vi "Generate Random Waveform.vi"(8 "error in":errorcluster, 11 "WaveformGen Settings":T1(array[cluster])) -> (0 "error out":errorcluster, 3 "Waveforms":waveform(dbl)[](array[waveform]))   [LabVIEW 2014]
uses:
  <userlib>/_OpenG.lib/numeric/numeric.llb/Random Number Within Range - DBL__ogtk.vi
  <vilib>/measure/NI_MABase.lvlib
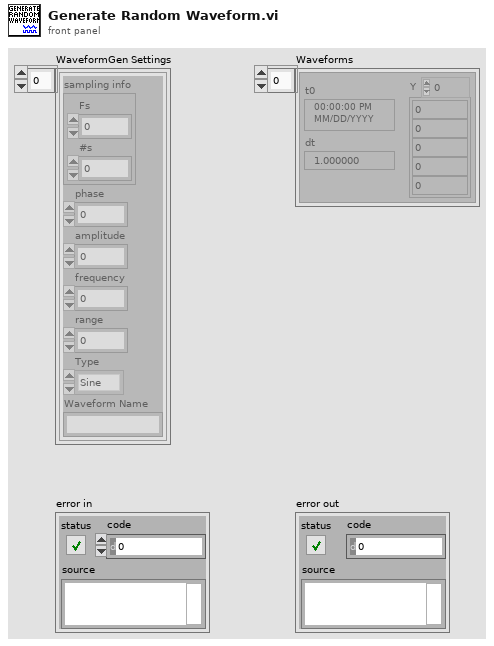
[diagram p1: front panel]
types:
  T1 = cluster{"sampling info":cluster{"Fs":dbl, "#s":dbl}, "phase":dbl, "amplitude":dbl, "frequency":dbl, "range":dbl, "Type":enum16{"Sine", "Triangle", "Sawtooth", "Square"}, "Waveform Name":string}[]
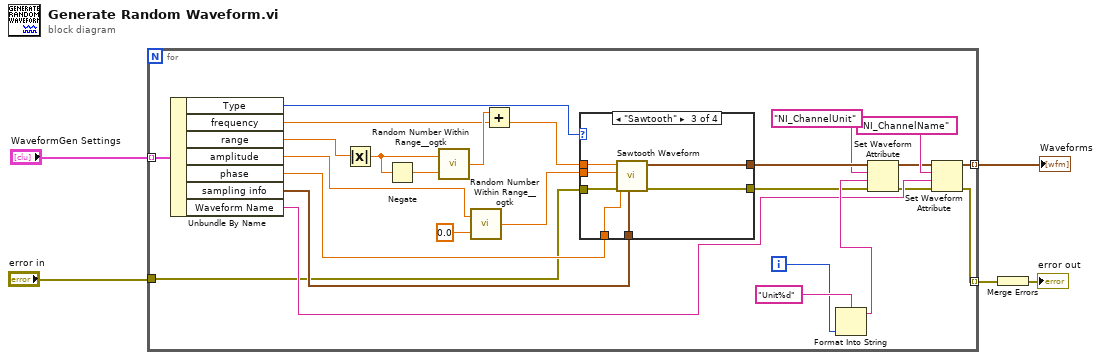
[diagram p0: block diagram]
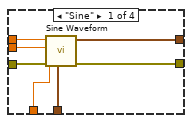
[diagram p2: hidden frame]
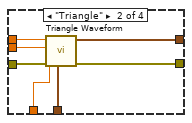
[diagram p3: hidden frame]
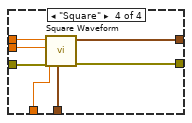
[diagram p4: hidden frame]
diagram:
  n1 = for {
    tunnel: "WaveformGen Settings" -> [w31] mode=indexing
    tunnel: [w21] -> w4 mode=indexing
    tunnel: [w7] -> w3 mode=indexing
    tunnel: "error in" -> [w6]
    i -> [w13]
    n2 = Unbundle By Name(w31) -> ("Type"=w11:enum16{"Sine", "Triangle", "Sawtooth", "Square"}, "frequency"=w25:dbl, "range"=w26:dbl, "amplitude"=w20:dbl, "phase"=w24:dbl, "sampling info"=w23:cluster{"Fs":dbl, "#s":dbl}, "Waveform Name"=w10:string)
    n3 = Absolute Value(x=w26) -> (abs(x)=w28:dbl)
    n4 = Negate(x=w28) -> (-x=w27:dbl)
    n5 = call-poly <userlib>:"Random Number Within Range__ogtk.vi"("High"=w28, "Low"=w27) -> ("Random Number"=w29:dbl)  [unwired: 3 in]
    n6 = call-poly <userlib>:"Random Number Within Range__ogtk.vi"("High"=w20, "Low"=0.0) -> ("Random Number"=w18:dbl)  [unwired: 3 in]
    n7 = Add(x=w29, y=w25) -> (x+y=w30:dbl)
    n8 = case shown="\"Sawtooth\"" w11 {
      tunnel: w30 -> [w38 w45 w52 w59]
      tunnel: w24 -> [w37 w44 w51 w58]
      tunnel: w23 -> [w36 w43 w50 w57]
      tunnel: w18 -> [w35 w42 w49 w56]
      tunnel: [w34 w41 w48 w55] -> w17
      tunnel: [w33 w40 w47 w53] -> w9
      tunnel: w6 -> [w32 w39 w46 w54]
      frame "Sine" {
        n9 = call <vilib>:"Sine Waveform.vi"("sampling info"=w36, "error in (no error)"=w32, "phase"=w37, "amplitude"=w35, "frequency"=w38) -> ("error out"=w33:errorcluster, "signal out"=w34:waveform(dbl))  [unwired: 5 in]
      }
      frame "Triangle" {
        n10 = call <vilib>:"Triangle Waveform.vi"("sampling info"=w43, "error in (no error)"=w39, "phase"=w44, "amplitude"=w42, "frequency"=w45) -> ("error out"=w40:errorcluster, "signal out"=w41:waveform(dbl))  [unwired: 5 in]
      }
      frame "Sawtooth" {
        n11 = call <vilib>:"Sawtooth Waveform.vi"("sampling info"=w50, "error in (no error)"=w46, "phase"=w51, "amplitude"=w49, "frequency"=w52) -> ("error out"=w47:errorcluster, "signal out"=w48:waveform(dbl))  [unwired: 5 in]
      }
      frame "Square" {
        n12 = call <vilib>:"Square Waveform.vi"("sampling info"=w57, "error in (no error)"=w54, "phase"=w58, "amplitude"=w56, "frequency"=w59) -> ("error out"=w53:errorcluster, "signal out"=w55:waveform(dbl))  [unwired: 5 in]
      }
    }
    n13 = Format Into String(format string="Unit%d" ("name"), w13) -> (resulting string=w12:string)  [unwired: 2 in, 1 out]
    n14 = Set Waveform Attribute(4:w9, 5:w12, 6:"NI_ChannelUnit" ("name"), 7:w17) -> (0:w8:errorcluster, 3:w16:waveform(dbl))  [unwired: 1 out]
    n15 = Set Waveform Attribute(4:w8, 5:w10, 6:"NI_ChannelName" ("name"), 7:w16) -> (0:w7:errorcluster, 3:w21:waveform(dbl))  [unwired: 1 out]
  }
  "Waveforms" <- w4
  n16 = Merge Errors(w3) -> (→"error out":errorcluster)
